vi "LabvolutionSubmoduleCheck_Provider_Shutdown.vi"(10 "Is Exiting":bool, 11 "reference":refnum<vi>) -> ()   [LabVIEW 2018]
panel:
  out "error out":errorcluster
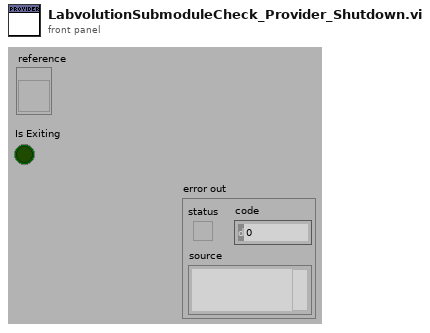
[diagram p1: front panel]
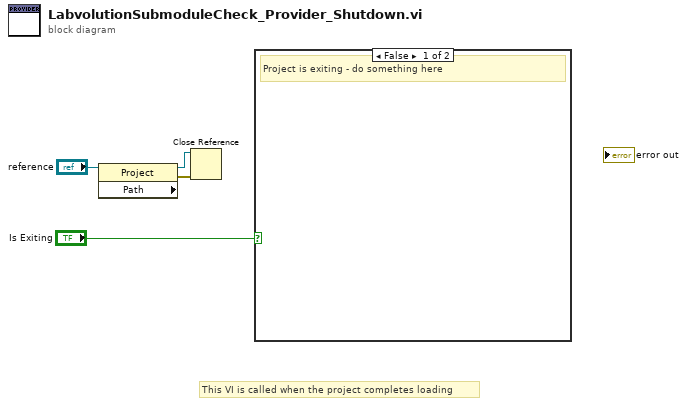
[diagram p0: block diagram]
diagram:
  # "This VI is called when the project completes loading"
  n1 = property class="Project" props=["Path"](reference="reference") -> (reference out=w2:refnum<vi>, error out=w3:errorcluster)  [unwired: 1 in, 1 out]
  n2 = Close Reference(reference=w2, error in (no error)=w3) -> ()  [unwired: 1 out]
  n3 = case shown="False" "Is Exiting" {
    frame False {
      # "Project is exiting - do something here"
    }
    frame True {
      # "LabVIEW is exiting - do nothing"
    }
  }
